vi "StopSweep.vi"(11 "FPGA in":refnum<queue>) -> (3 "FPGA out":refnum<queue>)   [LabVIEW 2019, in "FPGA.lvlib"]
uses:
  FPGA.lvlib
  FPGA.ctl
  Commands.ctl
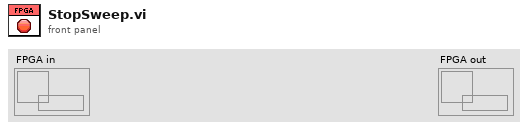
[diagram p1: front panel]
types:
  T1 = typedef "FPGA.lvlib/FPGA.ctl" = cluster{"Start freq. [Hz]":dbl, "Sweep duration [s]":dbl, "Freq. step [Hz]":dbl, "DAC Sample Rate":dbl, "ADC Sample Rate":dbl, "CMD port":u16, "DFAST port":u16, "CMD ID":refnum<k16>, "DFAST ID":refnum<k16>, "CMD error out":errorcluster, "FPGA IP":string, "DFAST error out ":errorcluster, "Stop freq. [Hz]":dbl, "Discrete sweep":bool, "Initial NCO":u32, "Difference NCO":i32, "step NCO":i64, "Final NCO":u32, "clocks for step":u32, "demodulation":bool, "NCO Phase Precision":u32, "NCO Sample Rate":dbl, "Time for step [s]":dbl, "NCO freq. resolution":dbl, "Sweep speed [Hz/s]":dbl, "Connected":bool, "Slew Rate [V/us]":dbl, "Parameters_ok":bool, "Amplitude [mVpp]":dbl, "Scale Factor":fxp<+,16,0>, "Acquiring":bool, "DAC-ADC Latency":u16, "Digital Gain":i32, "Number of steps":i32, "Averaging preferred":bool, "Filter Order":u32, "Settling":enum16{"99%", "99,9%"}}
  T2 = typedef "FPGA.lvlib/Commands.ctl" = string
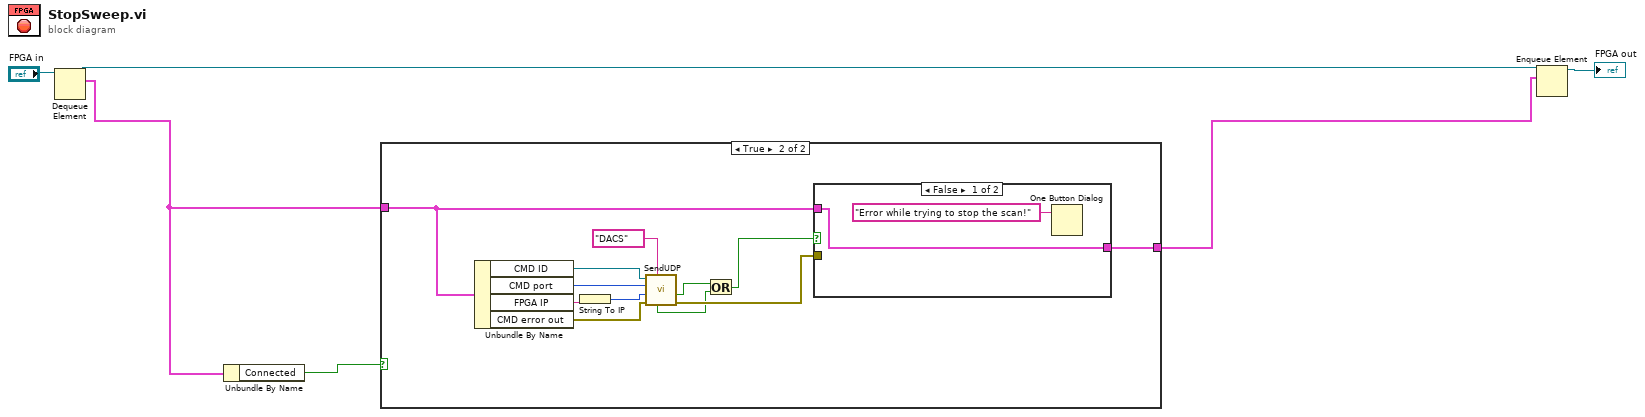
[diagram p0: block diagram]
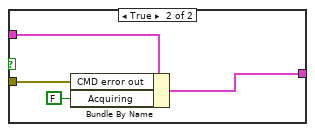
[diagram p3: hidden frame]
diagram:
  n1 = Dequeue Element(queue="FPGA in") -> (queue out=w5:refnum<queue>, element=w3:T1)  [unwired: 2 in, 2 out]
  n2 = Unbundle By Name(w3) -> ("Connected"=w1:bool)
  n3 = case shown="True" w1 {
    tunnel: w3 -> [w7 w18]
    tunnel: [w7 w17] -> w2
    frame False {
    }
    frame True {
      n4 = Unbundle By Name(w18) -> ("CMD ID"=w16:refnum<k16>, "CMD port"=w15:u16, "FPGA IP"=w19:string, "CMD error out"=w13:errorcluster)
      n5 = String To IP(1:w19) -> (0:w14:u32)
      n6 = call "SendUDP.vi"("data in"=T2 "DACS" ("Combo Box"), "error in (no error)"=w13, "address"=w14, "port or service name"=w15, "connection ID"=w16) -> ("error out"=w12:errorcluster, "ACK"=w10:bool, "ERR"=w9:bool)  [unwired: 1 in, 3 out]
      n7 = Or(x=w10, y=w9) -> (x .or. y?=w8:bool)
      n8 = case shown="False" w8 {
        tunnel: w18 -> [w20 w25]
        tunnel: [w20 w24] -> w17
        tunnel: w12 -> [_ w23]
        frame False {
          n9 = One Button Dialog(message="Error while trying to stop the scan!") -> ()  [unwired: 1 in, 1 out]
        }
        frame True {
          n10 = Bundle By Name(cluster=w25, "CMD error out"=w23, "Acquiring"=FALSE) -> (w24:T1)
        }
      }
    }
  }
  n11 = Enqueue Element(queue=w5, element=w2) -> (queue out=→"FPGA out":refnum<queue>)  [unwired: 2 in, 2 out]
